vi "Get Bricks Positions.vi"(8 "error in (no error)":errorcluster, 11 "object in":refnum<class "Wall.lvclass">) -> (0 "error out":errorcluster, 2 "Brick Wall":T1[](array[typedef]), 3 "object out":refnum<class "Wall.lvclass">)   [LabVIEW 2017, in "Wall.lvclass"]
uses:
  Wall.lvclass
  Controls/Coordinates.ctl
  Wall.lvclass/Wall.ctl
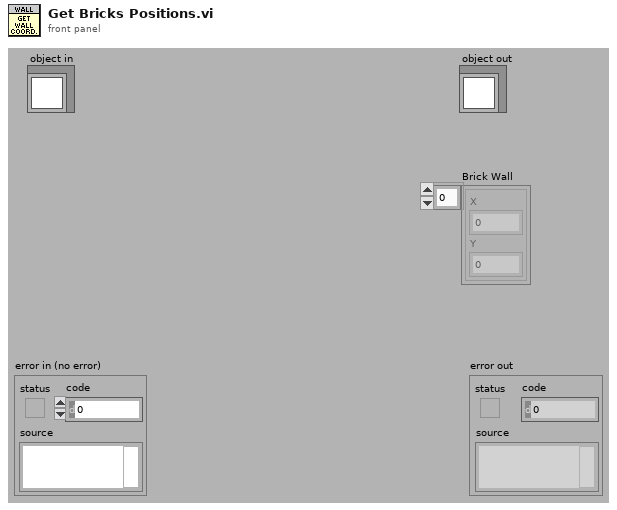
[diagram p1: front panel]
types:
  T1 = typedef "Coordinates.ctl" = cluster{"X":i32, "Y":i32}
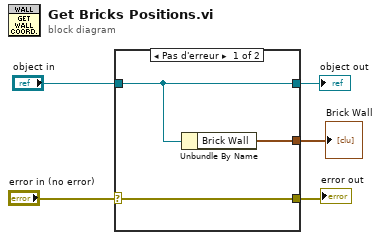
[diagram p0: block diagram]
diagram:
  n1 = case shown="Pas d'erreur" "error in (no error)" {
    selector: "error in (no error)" -> [w8 w10]
    tunnel: [w8 w10] -> w4
    tunnel: [w7 w9] -> w2
    tunnel: "object in" -> [w7 w9]
    tunnel: [w6 _] -> w1
    frame No Error {
      n2 = Unbundle By Name(w7) -> ("Brick Wall"=w6:T1[])
    }
    frame Error {
    }
  }
  "error out" <- w4
  "object out" <- w2
  "Brick Wall" <- w1
